vi "Duplicate Test.vi"() -> ()   [LabVIEW 2019, in "Test Executive.lvlib"]
uses:
  <vilib>/gpm_packages/@cs/test-executive/Source/Test Executive/TestExecutive/Test Executive.lvclass
  C:/Program Files/National Instruments/LabVIEW 2019/vi.lib/gpm_packages/@cs/test-executive/Source/Test Executive/ITestExecutive/ITest Executive.lvclass
  <vilib>/gpm_packages/@cs/test-executive/Source/Test Executive/Executioner/Executioner.lvclass
  <vilib>/gpm_packages/@cs/run-time-assertions/Source/Assert Equal/Assert Equal.lvclass
  C:/Program Files/National Instruments/LabVIEW 2019/vi.lib/gpm_packages/@cs/run-time-assertions/Source/Assert/Assert.lvclass
  3f58f81d-24f4-4b38-8029-ea7739ca710f.vi
  4ea763fe-e262-4f1b-8a79-0ca79b847688.vi
  6a21370e-3cef-4ac3-8829-bf63652873b0.vi
  103630d6-5241-4d15-b3ff-21d61f4a4c4c.vi
  36607b50-8362-4d71-bcc6-c0885ffd9225.vi
  <vilib>/Utility/error.llb/Error Cluster From Error Code.vi
  <vilib>/gpm_packages/@cs/test-executive/Source/Test Executive/ITestExecutive/ITest Executive.lvclass
  <vilib>/gpm_packages/@cs/test-executive/Source/Test Executive/Test Executive.lvlib
  <vilib>/gpm_packages/@cs/test-executive/Source/Test Executive/TestExecutive Ref/TestExecutive Ref.lvclass
panel:
  out "Root Names":string[](array[string])
  out "Root IDs":string[](array[string])
  in  "Tree Post Copy":string(tree)
  in  "Tree":string(tree)
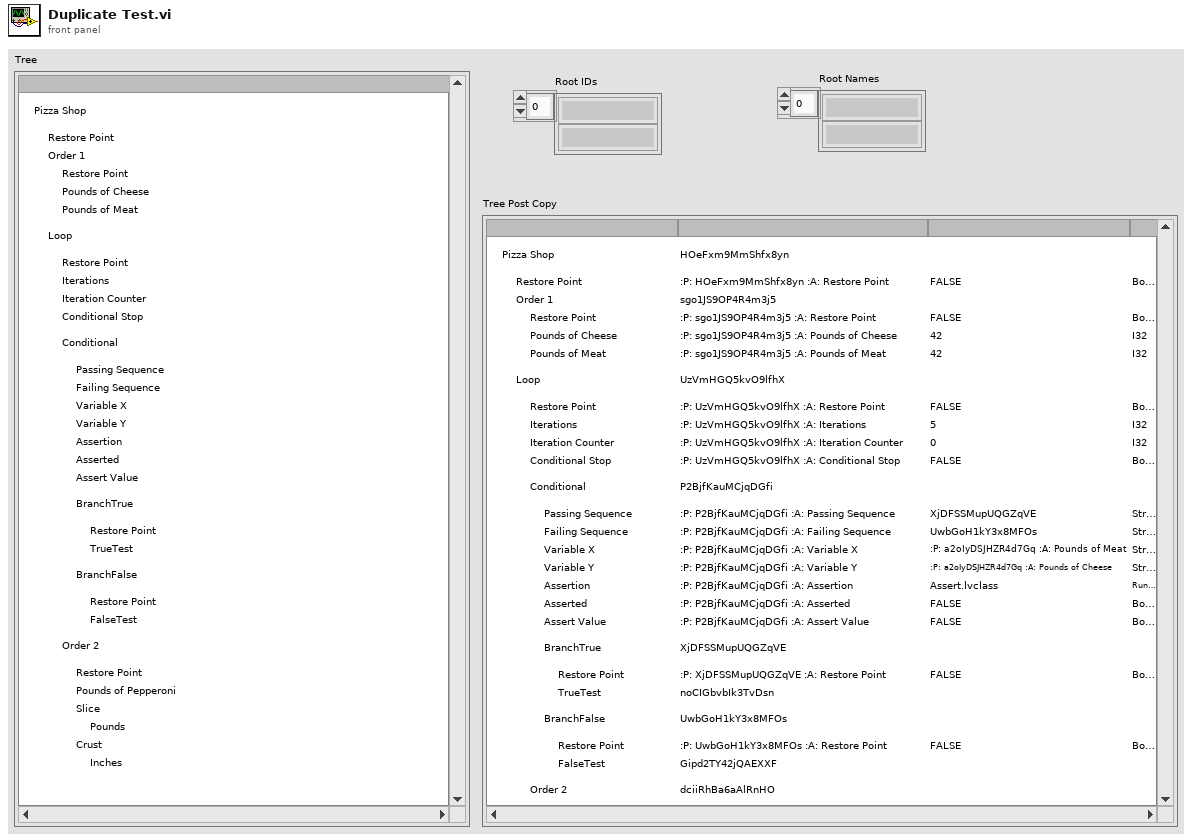
[diagram p1: front panel]
types:
  T1 = cluster{"Left Cell String":string, "Child Text":string[], "Child Tag":string, "Item Indent":i32, "Child Only?":bool, "Glyph Index":i32}[]
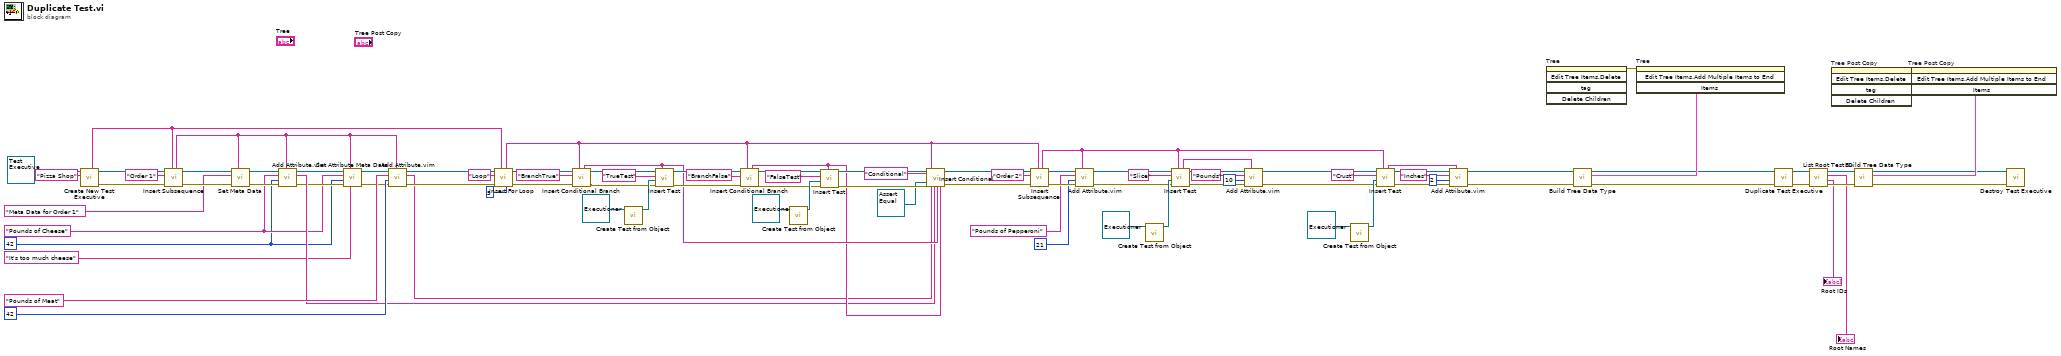
[diagram p0: block diagram]
diagram:
  w10 = 42
  w11 = "Pounds of Cheese" ("Attribute Name")
  n1 = call <vilib>:"Create New Test Executive.vi"("Name"="Pizza Shop", "Test Executive"=refnum<class "Test Executive.lvclass"> refnum ("Test Executive.lvlib:Test Executive.lvclass")) -> ("error out"=w87:errorcluster, "Test Executive Ref"=w88:refnum<data-value>, "Test Executive ID out"=w68:string)  [unwired: 7 in]
  n2 = call <vilib>:"Insert Subsequence.vi"("Parent ID"=w68, "error in (no error)"=w87, "Name"="Order 1", "Test Executive Ref"=w88) -> ("error out"=w20:errorcluster, "Test Executive Ref out"=w22:refnum<data-value>, "Unique ID out"=w12:string)  [unwired: 4 in, 1 out]
  n3 = call <vilib>:"Set Meta Data.vi"("Unique ID"=w12, "error in (no error)"=w20, "Meta Data"="Meta Data for Order 1", "Test Executive Ref"=w22) -> ("error out"=w19:errorcluster, "Test Executive Ref out"=w21:refnum<data-value>)  [unwired: 6 in]
  n4 = call "Add Attribute.vim"("ID"=w12, "error in (no error)"=w19, "Attribute"=w10, "Attribute Name"=w11, "Test Executive Ref"=w21) -> ("error out"=w14:errorcluster, "Attribute ID out"=w17:string, "Test Executive Ref out"=w16:refnum<data-value>)  [unwired: 3 in, 1 out]
  n5 = call <vilib>:"Set Attribute Meta Data.vi"("Meta Data"="It's too much cheese", "Unique ID"=w12, "error in (no error)"=w14, "Attribute Type"=w10, "Attribute Name"=w11, "Test Executive Ref"=w16) -> ("error out"=w13:errorcluster, "Test Executive Ref out"=w15:refnum<data-value>)  [unwired: 3 in, 1 out]
  n6 = call "Add Attribute.vim"("ID"=w12, "error in (no error)"=w13, "Attribute"=42, "Attribute Name"="Pounds of Meat", "Test Executive Ref"=w15) -> ("error out"=w26:errorcluster, "Attribute ID out"=w23:string, "Test Executive Ref out"=w27:refnum<data-value>)  [unwired: 3 in, 1 out]
  n7 = call <vilib>:"Insert For Loop.vi"("Loop Iterations"=5, "Parent ID"=w68, "error in (no error)"=w26, "Name"="Loop", "Test Executive Ref"=w27) -> ("error out"=w32:errorcluster, "Test Executive Ref out"=w34:refnum<data-value>, "Unique ID out"=w30:string)  [unwired: 3 in, 1 out]
  n8 = call <vilib>:"Insert Conditional Branch.vi"("Parent ID"=w30, "error in (no error)"=w32, "Name"="BranchTrue", "Test Executive Ref"=w34) -> ("error out"=w48:errorcluster, "Test Executive Ref out"=w47:refnum<data-value>, "Unique ID out"=w29:string)  [unwired: 4 in, 1 out]
  n9 = call <vilib>:"Create Test from Object.vi"("Test"=refnum<class "Executioner.lvclass"> refnum ("Test Executive.lvlib:Executioner.lvclass")) -> ("Test"=w49:refnum<class "Executioner.lvclass">)  [unwired: 10 in]
  n10 = call <vilib>:"Insert Test.vi"("Parent ID"=w29, "error in (no error)"=w48, "Test"=w49, "Name"="TrueTest", "Test Executive Ref"=w47) -> ("error out"=w41:errorcluster, "Test Executive Ref out"=w40:refnum<data-value>)  [unwired: 3 in, 2 out]
  n11 = call <vilib>:"Insert Conditional Branch.vi"("Parent ID"=w30, "error in (no error)"=w41, "Name"="BranchFalse", "Test Executive Ref"=w40) -> ("error out"=w43:errorcluster, "Test Executive Ref out"=w42:refnum<data-value>, "Unique ID out"=w28:string)  [unwired: 4 in, 1 out]
  n12 = call <vilib>:"Create Test from Object.vi"("Test"=refnum<class "Executioner.lvclass"> refnum ("Test Executive.lvlib:Executioner.lvclass")) -> ("Test"=w44:refnum<class "Executioner.lvclass">)  [unwired: 10 in]
  n13 = call <vilib>:"Insert Test.vi"("Parent ID"=w28, "error in (no error)"=w43, "Test"=w44, "Name"="FalseTest", "Test Executive Ref"=w42) -> ("error out"=w38:errorcluster, "Test Executive Ref out"=w37:refnum<data-value>)  [unwired: 3 in, 2 out]
  n14 = call <vilib>:"Insert Conditional.vi"("Test Executive Ref"=w37, "Name"="Conditional", "Assertion"=refnum<class "Assert Equal.lvclass"> refnum ("Run Time Assertions.lvlib:Assert Equal.lvclass"), "error in (no error)"=w38, "Parent ID"=w30, "Variable X"=w23, "Variable Y"=w17, "Passing Executive"=w29, "Failing Executive"=w28) -> ("Test Executive Ref out"=w33:refnum<data-value>, "error out"=w31:errorcluster)  [unwired: 7 in, 2 out]
  n15 = call <vilib>:"Insert Subsequence.vi"("Parent ID"=w30, "error in (no error)"=w31, "Name"="Order 2", "Test Executive Ref"=w33) -> ("error out"=w85:errorcluster, "Test Executive Ref out"=w84:refnum<data-value>, "Unique ID out"=w54:string)  [unwired: 4 in, 1 out]
  n16 = call "Add Attribute.vim"("ID"=w54, "error in (no error)"=w85, "Attribute"=21, "Attribute Name"="Pounds of Pepperoni", "Test Executive Ref"=w84) -> ("error out"=w71:errorcluster, "Test Executive Ref out"=w72:refnum<data-value>)  [unwired: 3 in, 2 out]
  n17 = call <vilib>:"Create Test from Object.vi"("Test"=refnum<class "Executioner.lvclass"> refnum ("Test Executive.lvlib:Executioner.lvclass")) -> ("Test"=w73:refnum<class "Executioner.lvclass">)  [unwired: 10 in]
  n18 = call <vilib>:"Insert Test.vi"("Parent ID"=w54, "error in (no error)"=w71, "Test"=w73, "Name"="Slice", "Test Executive Ref"=w72) -> ("error out"=w75:errorcluster, "Test Executive Ref out"=w79:refnum<data-value>, "Unique ID out"=w78:string)  [unwired: 3 in, 1 out]
  n19 = call "Add Attribute.vim"("ID"=w78, "error in (no error)"=w75, "Attribute"=10, "Attribute Name"="Pounds", "Test Executive Ref"=w79) -> ("error out"=w56:errorcluster, "Test Executive Ref out"=w58:refnum<data-value>)  [unwired: 3 in, 2 out]
  n20 = call <vilib>:"Create Test from Object.vi"("Test"=refnum<class "Executioner.lvclass"> refnum ("Test Executive.lvlib:Executioner.lvclass")) -> ("Test"=w65:refnum<class "Executioner.lvclass">)  [unwired: 10 in]
  n21 = call <vilib>:"Insert Test.vi"("Parent ID"=w54, "error in (no error)"=w56, "Test"=w65, "Name"="Crust", "Test Executive Ref"=w58) -> ("error out"=w63:errorcluster, "Test Executive Ref out"=w60:refnum<data-value>, "Unique ID out"=w53:string)  [unwired: 3 in, 1 out]
  n22 = call "Add Attribute.vim"("ID"=w53, "error in (no error)"=w63, "Attribute"=2, "Attribute Name"="Inches", "Test Executive Ref"=w60) -> ("error out"=w55:errorcluster, "Test Executive Ref out"=w57:refnum<data-value>)  [unwired: 3 in, 2 out]
  n23 = invoke on="Tree" class="Tree (strict)" method="Edit Tree Items.Delete"() -> (error out=w66:errorcluster)  [unwired: 5 in, 4 out]
  n24 = call <vilib>:"Build Tree Data Type.vi"("error in (no error)"=w55, "Test Executive Ref"=w57) -> ("error out"=w7:errorcluster, "Tree Data"=w67:T1, "Test Executive Ref out"=w8:refnum<data-value>)  [unwired: 7 in]
  n25 = invoke on="Tree" class="Tree (strict)" method="Edit Tree Items.Add Multiple Items to End"(error in=w66, "Items"=w67) -> ()  [unwired: 2 in, 4 out]
  n26 = call <vilib>:"Duplicate Test Executive.vi"("error in (no error)"=w7, "Test Executive Ref"=w8) -> ("error out"=w4:errorcluster, "Test Executive Ref out"=w6:refnum<data-value>)  [unwired: 7 in, 1 out]
  n27 = call <vilib>:"List Root Test ID.vi"("error in (no error)"=w4, "Test Executive Ref"=w6) -> ("error out"=w3:errorcluster, "Root IDs"=→"Root IDs":string[], "Root Names"=→"Root Names":string[], "Test Executive Ref out"=w5:refnum<data-value>)  [unwired: 5 in, 1 out]
  n28 = invoke on="Tree Post Copy" class="Tree (strict)" method="Edit Tree Items.Delete"() -> (error out=w91:errorcluster)  [unwired: 5 in, 4 out]
  n29 = call <vilib>:"Build Tree Data Type.vi"("error in (no error)"=w3, "Test Executive Ref"=w5) -> ("error out"=w89:errorcluster, "Tree Data"=w92:T1, "Test Executive Ref out"=w90:refnum<data-value>)  [unwired: 7 in]
  n30 = invoke on="Tree Post Copy" class="Tree (strict)" method="Edit Tree Items.Add Multiple Items to End"(error in=w91, "Items"=w92) -> ()  [unwired: 2 in, 4 out]
  n31 = call <vilib>:"Destroy Test Executive.vi"("error in (no error)"=w89, "Test Executive Ref"=w90) -> ()  [unwired: 9 in, 1 out]
